vi "Cockpit Data Loging ver5.vi"(9 "Serial Number":string="20311132013", 11 "Pass/Fail":bool) -> ()   [LabVIEW 2018]
uses:
  <vilib>/Utility/config.llb/Config Data RefNum.ctl
  <vilib>/Utility/config.llb/Read Key (U32).vi
  <vilib>/Utility/config.llb/Read Key (String).vi
  <vilib>/Utility/config.llb/NI_LVConfig.lvlib
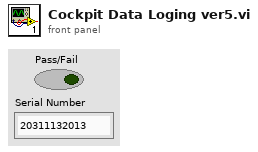
[diagram p1: front panel]
types:
  T1 = typedef "NI_LVConfig.lvlib/Config Data RefNum.ctl" = refnum<k1>
  T2 = cluster{"Base File Path":path, "Key Refnum":T1, "Shift":string, "Current Hour Actual":u32, "Shift Hour Data":u32[][], "Current Hour Index":i32, "Target Per Shift":u32, "Actual Per Shift":u32, "Reject":u32, "Target Per Week":u32, "Actual Per Week":u32, "FTT Target":u32, "Shift Number":u32, "Pass/Fail":bool, "Last Update Time":string, "Last Update Date":string, "Last Update Shift":string, "FTT Reject":u32, "Serial Number":string, "Serial Number Array":string[], "Last Update Week":string, "Week Shift Schedule":u32[], "FTT Percentage":u32, "Target Cummulative Per Shift":u32, "Target Cummulative Per Week":u32, "Target Cummulative Per Hour":u32}
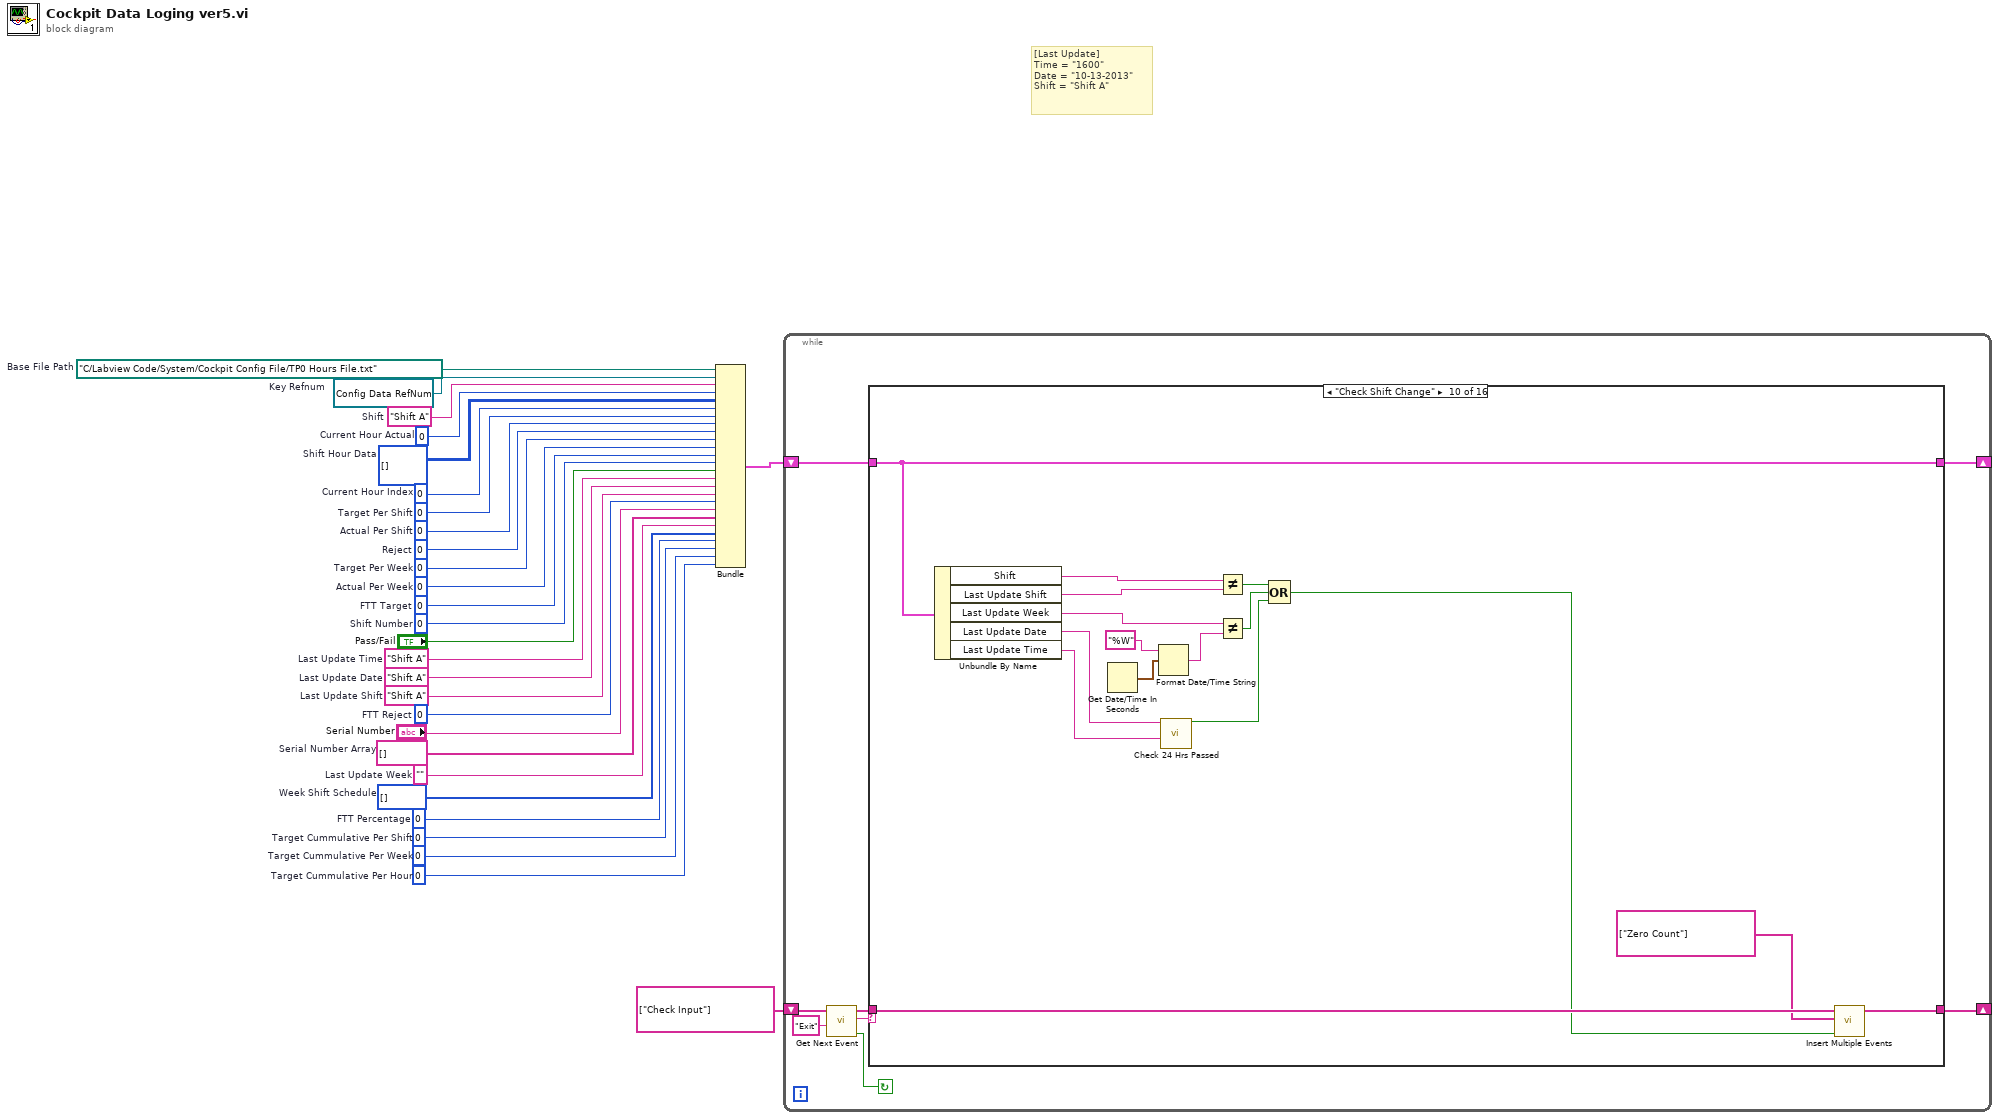
[diagram p0: block diagram]
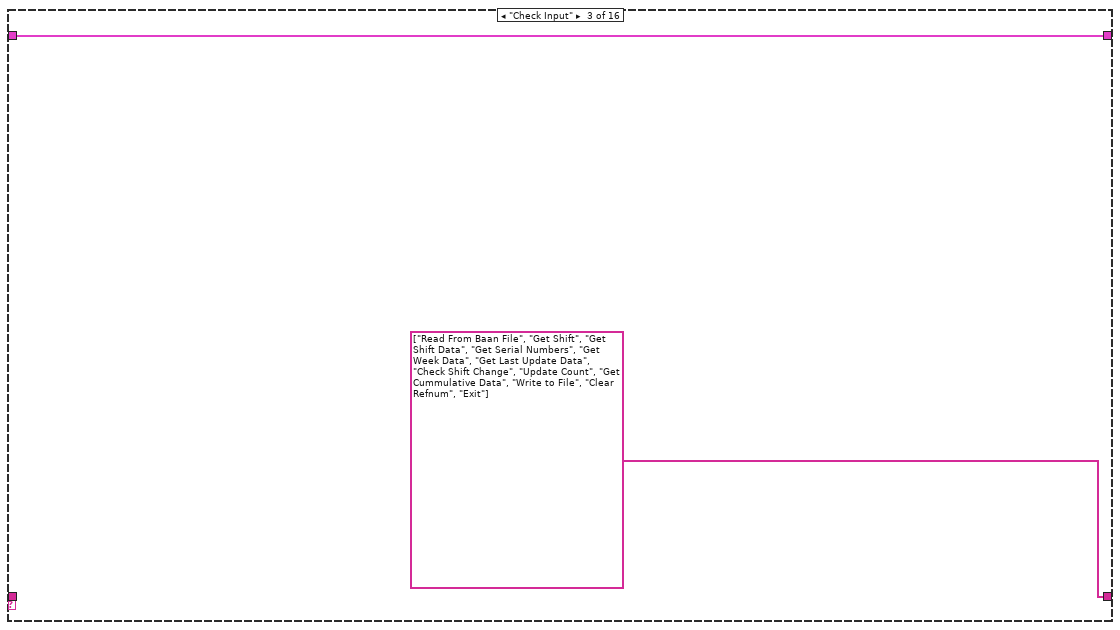
[diagram p4: hidden frame]
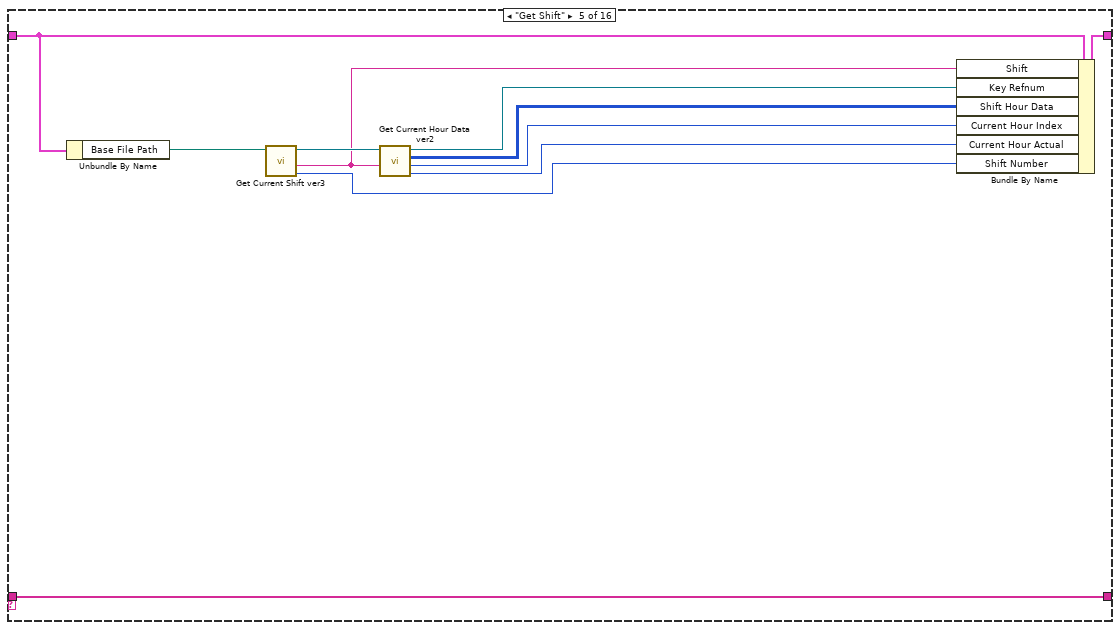
[diagram p6: hidden frame]
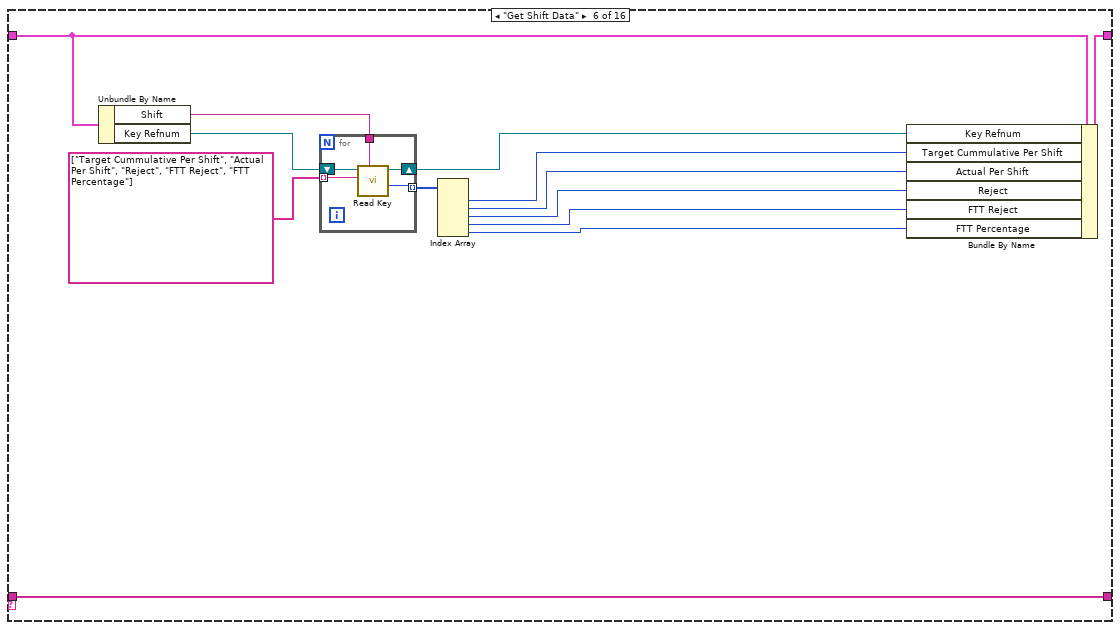
[diagram p7: hidden frame]
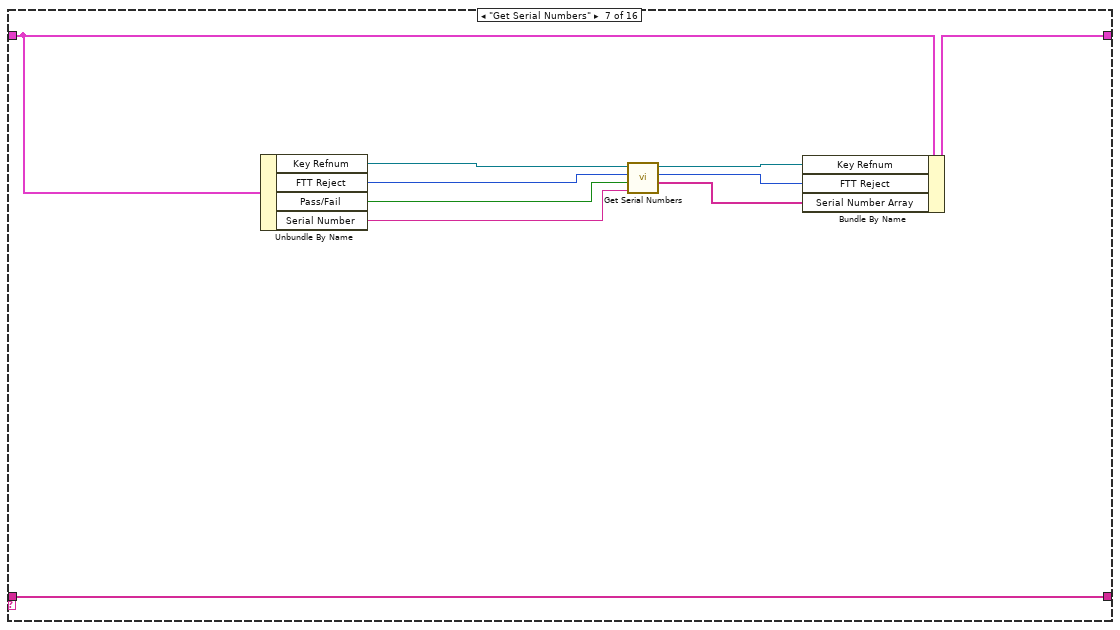
[diagram p8: hidden frame]
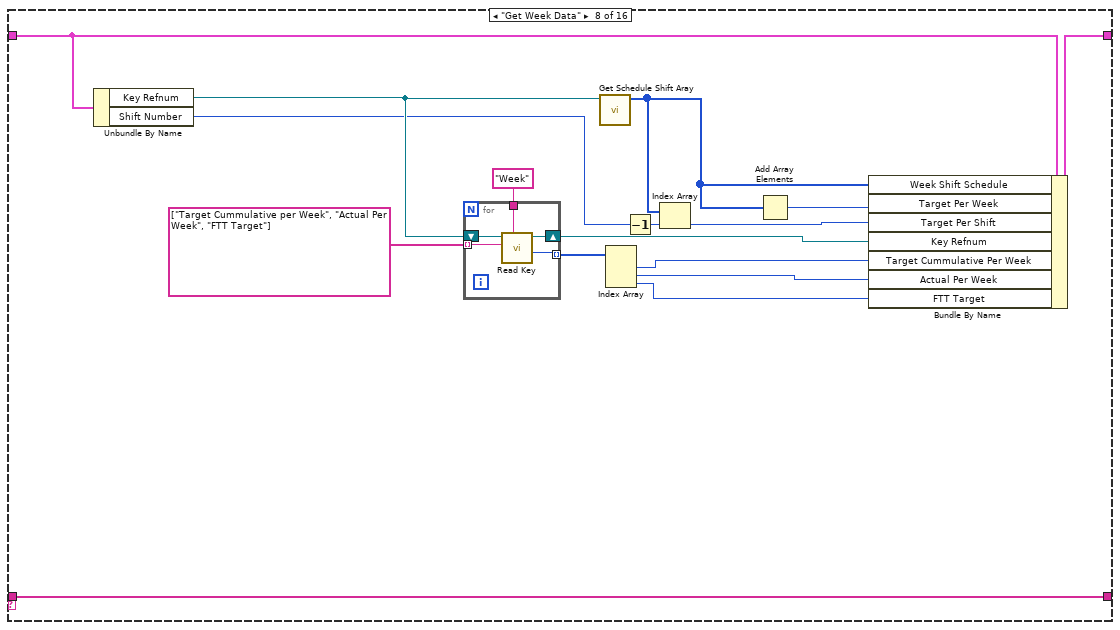
[diagram p9: hidden frame]
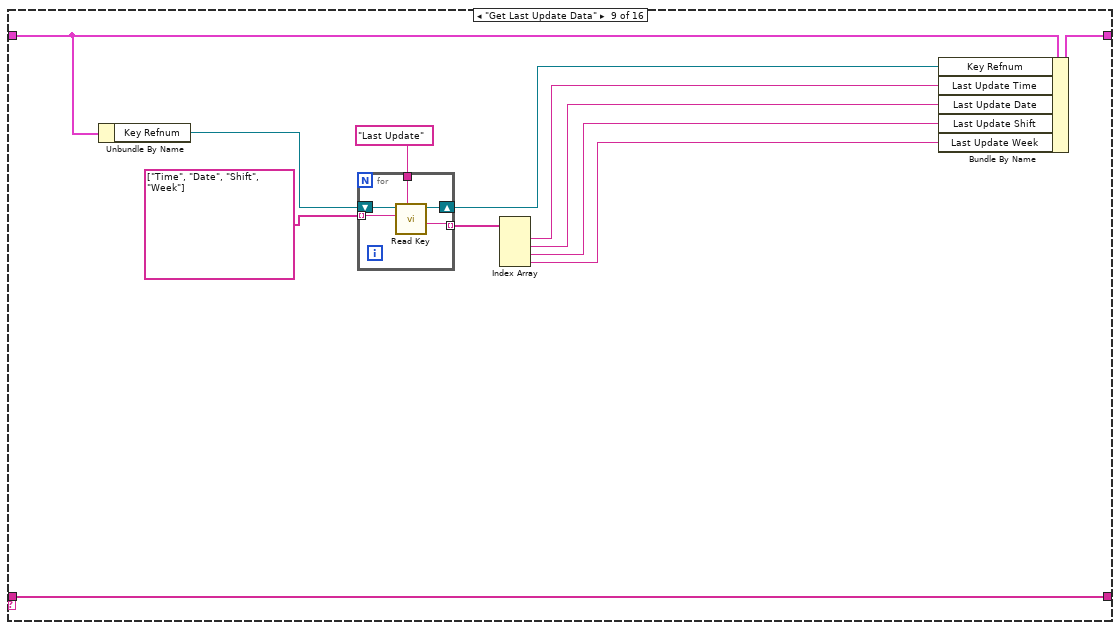
[diagram p10: hidden frame]
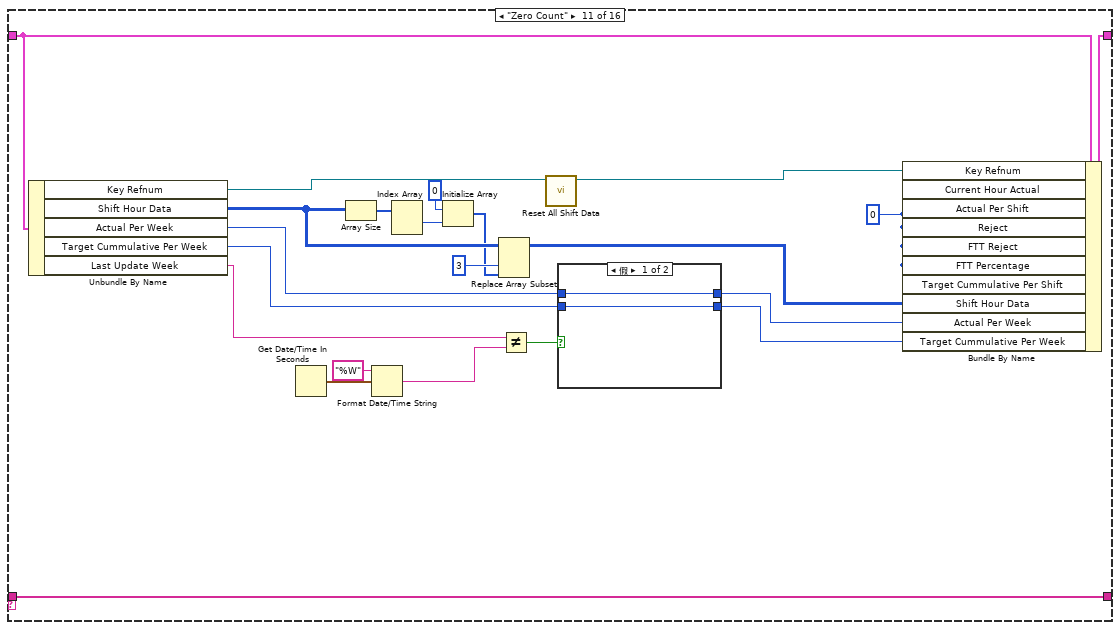
[diagram p11: hidden frame]
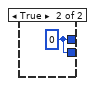
[diagram p12: hidden frame]
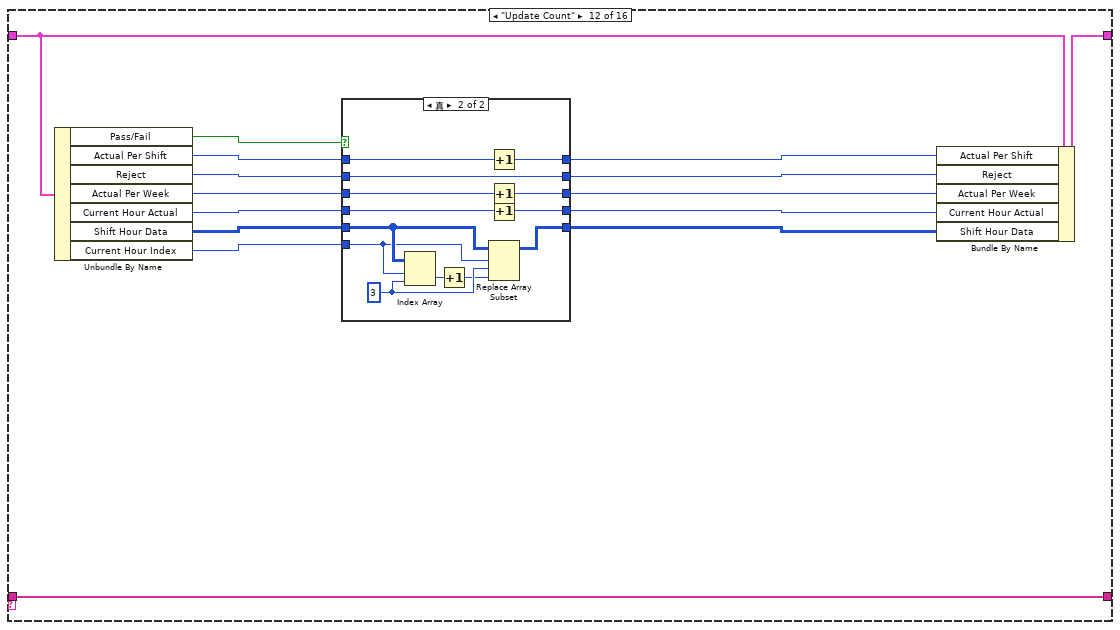
[diagram p13: hidden frame]
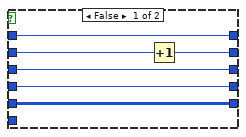
[diagram p14: hidden frame]
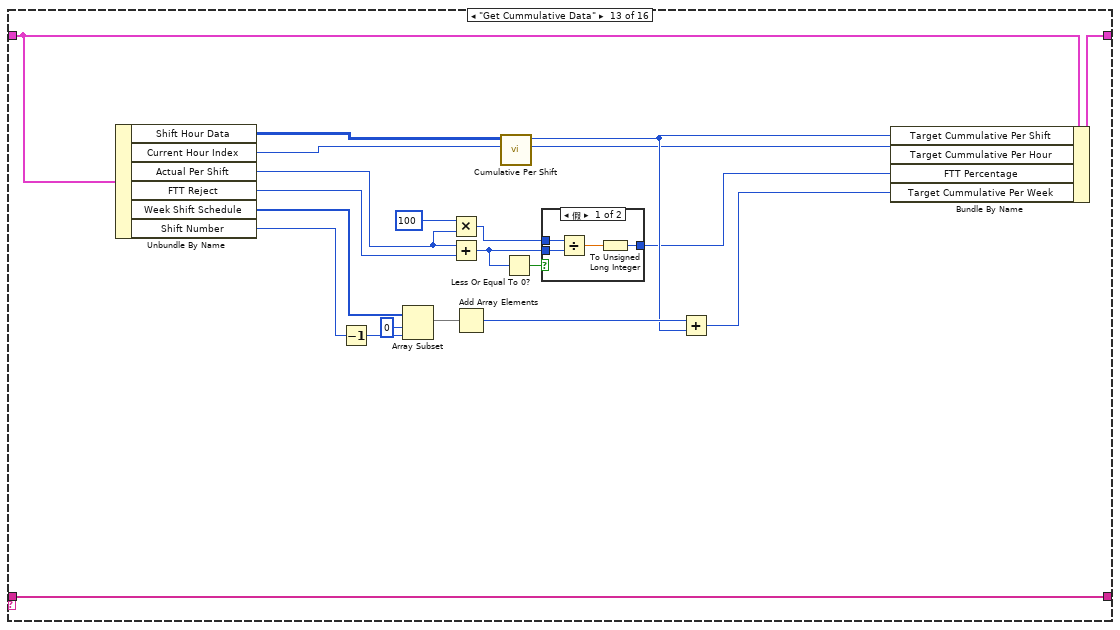
[diagram p15: hidden frame]
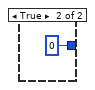
[diagram p16: hidden frame]
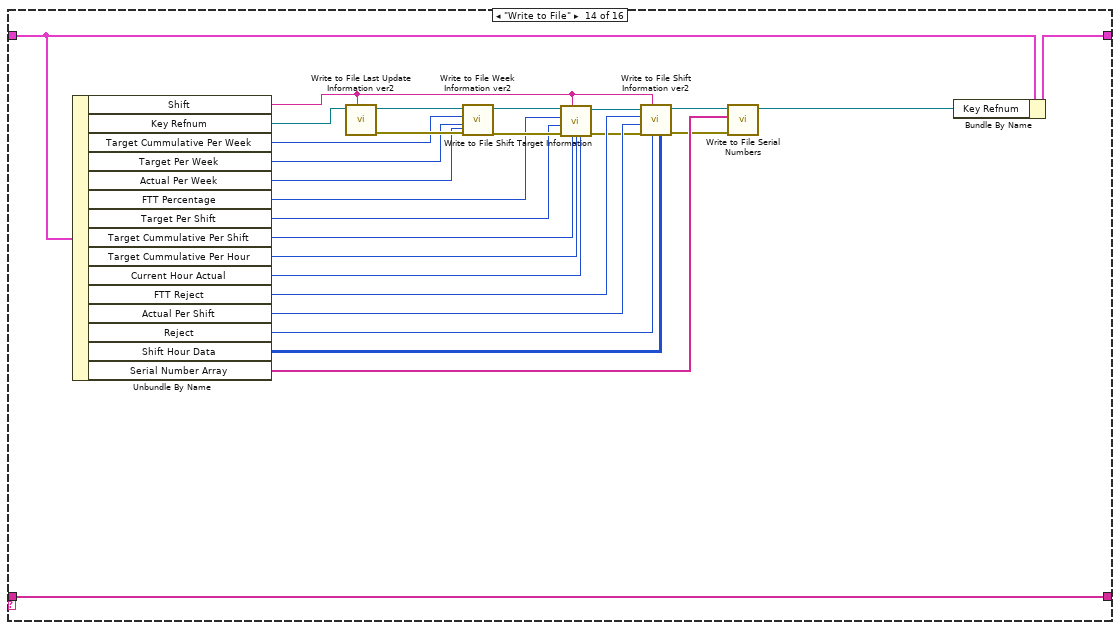
[diagram p17: hidden frame]
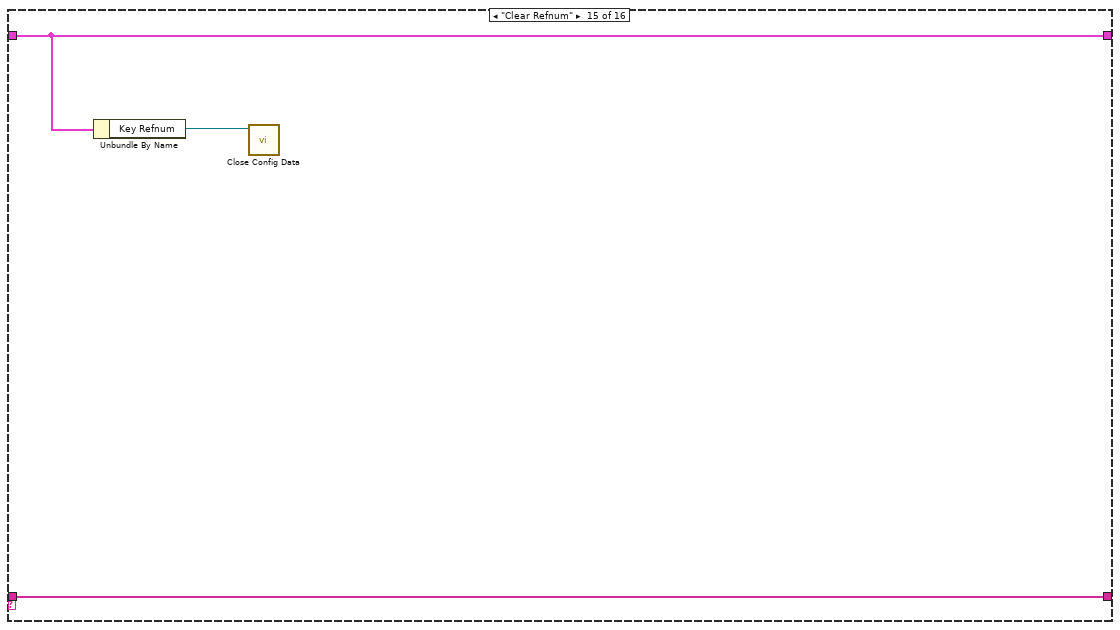
[diagram p18: hidden frame]
diagram:
  w1 = u32 0  # Target Cummulative Per Hour
  w2 = u32 0  # Target Cummulative Per Week
  w3 = u32 0  # Target Cummulative Per Shift
  w4 = u32 0  # FTT Percentage
  w5 = u32[] []  # Week Shift Schedule
  w6 = ""  # Last Update Week
  w7 = string[] []  # Serial Number Array
  w9 = u32 0  # FTT Reject
  w10 = "Shift A"  # Last Update Shift
  w11 = "Shift A"  # Last Update Date
  w12 = "Shift A"  # Last Update Time
  w14 = u32 0  # Shift Number
  w16 = u32 0  # Actual Per Week
  w17 = u32 0  # Target Per Week
  w15 = u32 0  # FTT Target
  w19 = u32 0  # Actual Per Shift
  w20 = u32 0  # Target Per Shift
  w18 = u32 0  # Reject
  w21 = 0  # Current Hour Index
  w22 = u32[][] []  # Shift Hour Data
  w23 = u32 0  # Current Hour Actual
  w24 = "Shift A"  # Shift
  w25 = T1 refnum items=["config data"]  # Key Refnum
  w27 = path "C:/Labview Code/System/Cockpit Config File/TP0 Hours File.txt"  # Base File Path
  # "[Last Update]\nTime = \"1600\"\nDate = \"10-13-2013\"\nShift = \"Shift A\""
  n1 = Bundle("Base File Path"=w27, "Key Refnum"=w25, "Shift"=w24, "Current Hour Actual"=w23, "Shift Hour Data"=w22, "Current Hour Index"=w21, "Target Per Shift"=w20, "Actual Per Shift"=w19, "Reject"=w18, "Target Per Week"=w17, "Actual Per Week"=w16, "FTT Target"=w15, "Shift Number"=w14, "Pass/Fail"="Pass/Fail", "Last Update Time"=w12, "Last Update Date"=w11, "Last Update Shift"=w10, "FTT Reject"=w9, "Serial Number"="Serial Number", "Serial Number Array"=w7, "Last Update Week"=w6, "Week Shift Schedule"=w5, "FTT Percentage"=w4, "Target Cummulative Per Shift"=w3, "Target Cummulative Per Week"=w2, "Target Cummulative Per Hour"=w1) -> (w26:T2)  [unwired: 1 in]
  n2 = while {
    shift-right: [w34] -> _
    shift-left: string[] ["Check Input"] ("event queue out") -> [w33]
    shift-right: [w31] -> _
    shift-left: w26 -> [w32]
    stop <- w30 continue-if-true
    n3 = call "Get Next Event.vi"("Exit Event"="Exit", "event queue in"=w33) -> ("Condition (Exit:F)"=w30:bool, "next event"=w35:string, "event queue out"=w36:string[])  [unwired: 3 in]
    n4 = case shown="\"Check Shift Change\"" w35 {
      tunnel: w36 -> [w38 w40 _ w44 w55 w68 w83 w99 w116 w130 w159 w177 w217 w249 w252 w253]
      tunnel: [w38 w40 string[] ["Read From Baan File", "Get Shift", "Get Shift Data", "Get Serial Numbers", "Get Week Data", "Get Last Update Data", "Check Shift Change", "Update Count", "Get Cummulative Data", "Write to File", "Clear Refnum", "Exit"] ("event queue out") w44 w55 w68 w83 w99 w116 w131 w159 w177 w217 w249 w252 w253] -> w34
      tunnel: w32 -> [w37 w39 w42 w43 w54 w63 w82 w98 w115 w137 w157 w176 w202 w248 w251 w254]
      tunnel: [w37 w39 w42 w43 w52 w62 w79 w97 w114 w137 w158 w168 w201 w240 w251 w254] -> w31
      frame "Error", Default {
      }
      frame "Init" {
      }
      frame "Check Input" {
      }
      frame "Read From Baan File" {
      }
      frame "Get Shift" {
        n5 = Unbundle By Name(w54) -> ("Base File Path"=w53:path)
        n6 = call "Get Current Shift ver3.vi"("Base File Path"=w53) -> ("Current Shift Number"=w45:u32, "Shift"=w49:string, "refnum out"=w51:T1)  [unwired: 7 in]
        n7 = call "Get Current Hour Data ver2.vi"("Shift"=w49, "Refnum in"=w51) -> ("Current Hour Actual"=w46:u32, "Hour Index"=w47:i32, "Shift Hour Data"=w48:u32[][], "Refnum Out"=w50:T1)  [unwired: 5 in, 1 out]
        n8 = Bundle By Name(cluster=w54, "Shift"=w49, "Key Refnum"=w50, "Shift Hour Data"=w48, "Current Hour Index"=w47, "Current Hour Actual"=w46, "Shift Number"=w45) -> (w52:T2)
      }
      frame "Get Shift Data" {
        n9 = Unbundle By Name(w63) -> ("Shift"=w65:string, "Key Refnum"=w64:T1)
        n10 = for {
          tunnel: string[] ["Target Cummulative Per Shift", "Actual Per Shift", "Reject", "FTT Reject", "FTT Percentage"] -> [w71] mode=indexing
          tunnel: w65 -> [w73]
          tunnel: [w70] -> w66 mode=indexing
          shift-right: [w69] -> w58
          shift-left: w64 -> [w72]
          n11 = call-poly <vilib>:"Read Key.vi"("section"=w73, "key"=w71, "refnum"=w72) -> ("value"=w70:u32, "refnum out"=w69:T1)  [unwired: 5 in, 2 out]
        }
        n12 = Index Array(array=w66) -> (element #1=w61:u32, element #2=w60:u32, element #3=w59:u32, element #4=w57:u32, element #5=w56:u32)  [unwired: 5 in]
        n13 = Bundle By Name(cluster=w63, "Key Refnum"=w58, "Target Cummulative Per Shift"=w61, "Actual Per Shift"=w60, "Reject"=w59, "FTT Reject"=w57, "FTT Percentage"=w56) -> (w62:T2)
      }
      frame "Get Serial Numbers" {
        n14 = Unbundle By Name(w82) -> ("Key Refnum"=w81:T1, "FTT Reject"=w75:u32, "Pass/Fail"=w80:bool, "Serial Number"=w74:string)
        n15 = call "Get Serial Numbers.vi"("Serial Number"=w74, "Pass/Fail"=w80, "FTT Reject in"=w75, "Refnum in"=w81) -> ("Array"=w78:string[], "FTT Reject out"=w77:u32, "Refnum out"=w76:T1)  [unwired: 5 in]
        n16 = Bundle By Name(cluster=w82, "Key Refnum"=w76, "FTT Reject"=w77, "Serial Number Array"=w78) -> (w79:T2)
      }
      frame "Get Week Data" {
        n17 = Unbundle By Name(w98) -> ("Key Refnum"=w89:T1, "Shift Number"=w85:u32)
        n18 = for {
          tunnel: string[] ["Target Cummulative per Week", "Actual Per Week", "FTT Target"] -> [w102] mode=indexing
          tunnel: "Week" ("Shift") -> [w104]
          tunnel: [w101] -> w95 mode=indexing
          shift-right: [w100] -> w90
          shift-left: w89 -> [w103]
          n19 = call-poly <vilib>:"Read Key.vi"("section"=w104, "key"=w102, "refnum"=w103) -> ("value"=w101:u32, "refnum out"=w100:T1)  [unwired: 5 in, 2 out]
        }
        n20 = call "Get Schedule Shift Aray.vi"("Refnum in"=w89) -> ("Array"=w86:u32[])  [unwired: 10 in]
        n21 = Index Array(array=w95) -> (element #1=w93:u32, element #2=w92:u32, element #3=w91:u32)  [unwired: 3 in]
        n22 = Decrement(x=w85) -> (x-1=w87:u32)
        n23 = Index Array(array=w86, index=w87) -> (element=w84:u32)
        n24 = Add Array Elements(numeric array=w86) -> (sum=w88:u32)
        n25 = Bundle By Name(cluster=w98, "Week Shift Schedule"=w86, "Target Per Week"=w88, "Target Per Shift"=w84, "Key Refnum"=w90, "Target Cummulative Per Week"=w93, "Actual Per Week"=w92, "FTT Target"=w91) -> (w97:T2)
      }
      frame "Get Last Update Data" {
        n26 = Unbundle By Name(w115) -> ("Key Refnum"=w110:T1)
        n27 = for {
          tunnel: string[] ["Time", "Date", "Shift", "Week"] -> [w119] mode=indexing
          tunnel: "Last Update" ("Shift") -> [w121]
          tunnel: [w118] -> w112 mode=indexing
          shift-right: [w117] -> w106
          shift-left: w110 -> [w120]
          n28 = call-poly <vilib>:"Read Key.vi"("section"=w121, "key"=w119, "refnum"=w120) -> ("value"=w118:string, "refnum out"=w117:T1)  [unwired: 5 in, 2 out]
        }
        n29 = Index Array(array=w112) -> (element #1=w109:string, element #2=w108:string, element #3=w107:string, element #4=w105:string)  [unwired: 4 in]
        n30 = Bundle By Name(cluster=w115, "Key Refnum"=w106, "Last Update Time"=w109, "Last Update Date"=w108, "Last Update Shift"=w107, "Last Update Week"=w105) -> (w114:T2)
      }
      frame "Check Shift Change" {
        n31 = Unbundle By Name(w137) -> ("Shift"=w136:string, "Last Update Shift"=w135:string, "Last Update Week"=w132:string, "Last Update Date"=w125:string, "Last Update Time"=w124:string)
        n32 = Get Date/Time In Seconds() -> (seconds since 1Jan1904=w134:timestamp)
        n33 = Format Date/Time String(time format string (%c)="%W", seconds (now)=w134) -> (date/time string=w133:string)  [unwired: 1 in]
        n34 = call "Check 24 Hrs Passed.vi"("Time String"=w124, "Date String"=w125) -> ("24 Hrs Passed?"=w123:bool)  [unwired: 9 in]
        n35 = Not Equal?(x=w136, y=w135) -> (x != y?=w127:bool)
        n36 = Not Equal?(x=w132, y=w133) -> (x != y?=w126:bool)
        n37 = Compound Arithmetic op=OR(w127, w126, w123) -> (w122:bool)
        n38 = call "Insert Multiple Events.vi"("Insert all? (T)"=w122, "Events to Insert"=string[] ["Zero Count"] ("event queue out"), "Event queue in"=w130) -> ("Event queue out"=w131:string[])  [unwired: 4 in]
      }
      frame "Zero Count" {
        w138 = u32 0 ("Current Hour Actual")
        n39 = Unbundle By Name(w157) -> ("Key Refnum"=w145:T1, "Shift Hour Data"=w154:u32[][], "Actual Per Week"=w148:u32, "Target Cummulative Per Week"=w140:u32, "Last Update Week"=w146:string)
        n40 = Get Date/Time In Seconds() -> (seconds since 1Jan1904=w149:timestamp)
        n41 = Array Size(array=w154) -> (size(s)=w156:i32[])
        n42 = Format Date/Time String(time format string (%c)="%W", seconds (now)=w149) -> (date/time string=w141:string)  [unwired: 1 in]
        n43 = Index Array(array=w156) -> (element #1=w143:i32)  [unwired: 2 in, 1 out]
        n44 = Initialize Array(u32 0 ("Current Hour Actual"), w143) -> (w152:u32[])
        n45 = Replace Array Subset(array=w154, new element=w152, index (col)=3 ("disabled index (col)")) -> (w151:u32[][])  [unwired: 1 in]
        n46 = Not Equal?(x=w146, y=w141) -> (x != y?=w142:bool)
        n47 = call "Reset All Shift Data.vi"("refnum in"=w145) -> ("refnum out"=w144:T1)  [unwired: 10 in]
        n48 = case shown="假" w142 {
          tunnel: w148 -> [w161 _]
          tunnel: [w161 w162] -> w147
          tunnel: w140 -> [w160 _]
          tunnel: [w160 w162] -> w139
          frame False {
          }
          frame True {
            w162 = u32 0 ("Actual Per Week")
          }
        }
        n49 = Bundle By Name(cluster=w157, "Key Refnum"=w144, "Current Hour Actual"=w138, "Actual Per Shift"=w138, "Reject"=w138, "FTT Reject"=w138, "FTT Percentage"=w138, "Target Cummulative Per Shift"=w138, "Shift Hour Data"=w151, "Actual Per Week"=w147, "Target Cummulative Per Week"=w139) -> (w158:T2)
      }
      frame "Update Count" {
        n50 = Unbundle By Name(w176) -> ("Pass/Fail"=w175:bool, "Actual Per Shift"=w174:u32, "Reject"=w173:u32, "Actual Per Week"=w172:u32, "Current Hour Actual"=w171:u32, "Shift Hour Data"=w170:u32[][], "Current Hour Index"=w169:i32)
        n51 = case shown="真" w175 {
          tunnel: w174 -> [w183 w196]
          tunnel: w173 -> [w182 w193]
          tunnel: w172 -> [w181 w195]
          tunnel: w171 -> [w180 w194]
          tunnel: w170 -> [w178 w189]
          tunnel: [w179 w193] -> w166
          tunnel: [w183 w192] -> w167
          tunnel: [w181 w191] -> w165
          tunnel: [w180 w190] -> w164
          tunnel: [w178 w185] -> w163
          tunnel: w169 -> [_ w187]
          frame False {
            n52 = Increment(x=w182) -> (x+1=w179:u32)
          }
          frame True {
            w186 = 3 ("disabled index (col)")
            n53 = Index Array(array=w189, index (row)=w187, index (col)=w186) -> (element=w188:u32)
            n54 = Increment(x=w188) -> (x+1=w184:u32)
            n55 = Increment(x=w196) -> (x+1=w192:u32)
            n56 = Increment(x=w195) -> (x+1=w191:u32)
            n57 = Increment(x=w194) -> (x+1=w190:u32)
            n58 = Replace Array Subset(array=w189, new element=w184, index (row)=w187, index (col)=w186) -> (w185:u32[][])
          }
        }
        n59 = Bundle By Name(cluster=w176, "Actual Per Shift"=w167, "Reject"=w166, "Actual Per Week"=w165, "Current Hour Actual"=w164, "Shift Hour Data"=w163) -> (w168:T2)
      }
      frame "Get Cummulative Data" {
        n60 = Unbundle By Name(w202) -> ("Shift Hour Data"=w205:u32[][], "Current Hour Index"=w204:i32, "Actual Per Shift"=w213:u32, "FTT Reject"=w216:u32, "Week Shift Schedule"=w212:u32[], "Shift Number"=w211:u32)
        n61 = Decrement(x=w211) -> (x-1=w203:u32)
        n62 = Array Subset(array=w212, index=0, length=w203) -> (w209:u32[])
        n63 = Multiply(x=u32 100 ("y"), y=w213) -> (x*y=w215:u32)
        n64 = Add(x=w213, y=w216) -> (x+y=w208:u32)
        n65 = Add Array Elements(numeric array=w209) -> (sum=w206:u32)
        n66 = call "Cumulative Per Shift.vi"("Current Hour Index"=w204, "Shift Hour Data"=w205) -> ("Target Cummulative Per Hour"=w197:u32, "Target Cummulative Per Shift"=w200:u32)  [unwired: 8 in]
        n67 = Less Or Equal To 0?(x=w208) -> (x <= 0?=w207:bool)
        n68 = case shown="假" w207 {
          tunnel: w215 -> [w221 _]
          tunnel: w208 -> [w219 _]
          tunnel: [w218 u32 0] -> w199
          frame False {
            n69 = Divide(x=w221, y=w219) -> (x/y=w220:dbl)
            n70 = To Unsigned Long Integer(number=w220) -> (unsigned 32bit integer=w218:u32)
          }
          frame True {
          }
        }
        n71 = Add(x=w206, y=w200) -> (x+y=w198:u32)
        n72 = Bundle By Name(cluster=w202, "Target Cummulative Per Shift"=w200, "Target Cummulative Per Hour"=w197, "FTT Percentage"=w199, "Target Cummulative Per Week"=w198) -> (w201:T2)
      }
      frame "Write to File" {
        n73 = Unbundle By Name(w248) -> ("Shift"=w231:string, "Key Refnum"=w247:T1, "Target Cummulative Per Week"=w235:u32, "Target Per Week"=w234:u32, "Actual Per Week"=w244:u32, "FTT Percentage"=w225:u32, "Target Per Shift"=w226:u32, "Target Cummulative Per Shift"=w227:u32, "Target Cummulative Per Hour"=w223:u32, "Current Hour Actual"=w224:u32, "FTT Reject"=w236:u32, "Actual Per Shift"=w243:u32, "Reject"=w242:u32, "Shift Hour Data"=w241:u32[][], "Serial Number Array"=w237:string[])
        n74 = call "Write to File Last Update Information ver2.vi"("Shift"=w231, "Refnum in"=w247) -> ("error out"=w245:errorcluster, "refnum out"=w246:T1)  [unwired: 8 in]
        n75 = call "Write to File Week Information ver2.vi"("Actual Per Week"=w244, "error in (no error)"=w245, "Target Per Week"=w234, "Target Cummulative Per Week"=w235, "Refnum in"=w246) -> ("error out"=w230:errorcluster, "Refnum out"=w233:T1)  [unwired: 5 in]
        n76 = call "Write to File Shift Target Information.vi"("Actual Per hour"=w224, "Target Cummulative Per Hour"=w223, "Target Cummulative Per Shift"=w227, "Shift"=w231, "error in"=w230, "Taregt Per Shift"=w226, "FTT Percentage"=w225, "Refnum in"=w233) -> ("error out"=w229:errorcluster, "refnum out"=w232:T1)  [unwired: 2 in]
        n77 = call "Write to File Shift Information ver2.vi"("Shift Hour Data"=w241, "Reject"=w242, "Shift"=w231, "error in"=w229, "Actual Per Shift"=w243, "FTT Reject"=w236, "Refnum in"=w232) -> ("error out"=w228:errorcluster, "refnum out"=w239:T1)  [unwired: 3 in]
        n78 = call "Write to File Serial Numbers.vi"("error in"=w228, "Serial Numbers Array"=w237, "Refnum in"=w239) -> ("refnum out"=w238:T1)  [unwired: 7 in, 1 out]
        n79 = Bundle By Name(cluster=w248, "Key Refnum"=w238) -> (w240:T2)
      }
      frame "Clear Refnum" {
        n80 = Unbundle By Name(w251) -> ("Key Refnum"=w250:T1)
        n81 = call <vilib>:"Close Config Data.vi"("refnum"=w250) -> ()  [unwired: 9 in, 2 out]
      }
      frame "Exit" {
      }
    }
  }
